vi "TCP - Client.vi"() -> ()   [LabVIEW 2023]
doc: "Demonstrates how to open a connection to an TCP server, read the data being sent, and display the data on a chart. This VI is designed to stop if the TCP connection is terminated."
panel:
  out "X4":bool
  out "X2":bool
  out "X3":bool
  out "X1":bool
  out "Switch 1":bool
  out "Switch 2":bool
  out "data out":string
  in  "Stop":bool
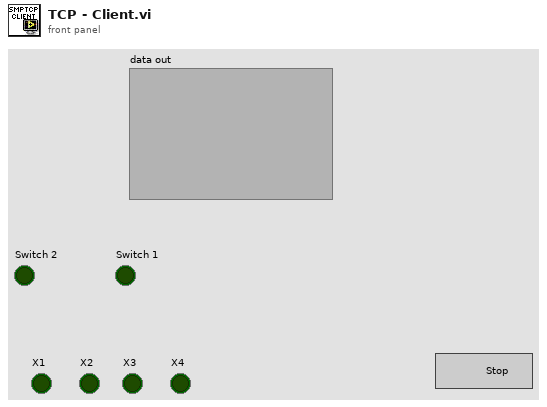
[diagram p1: front panel]
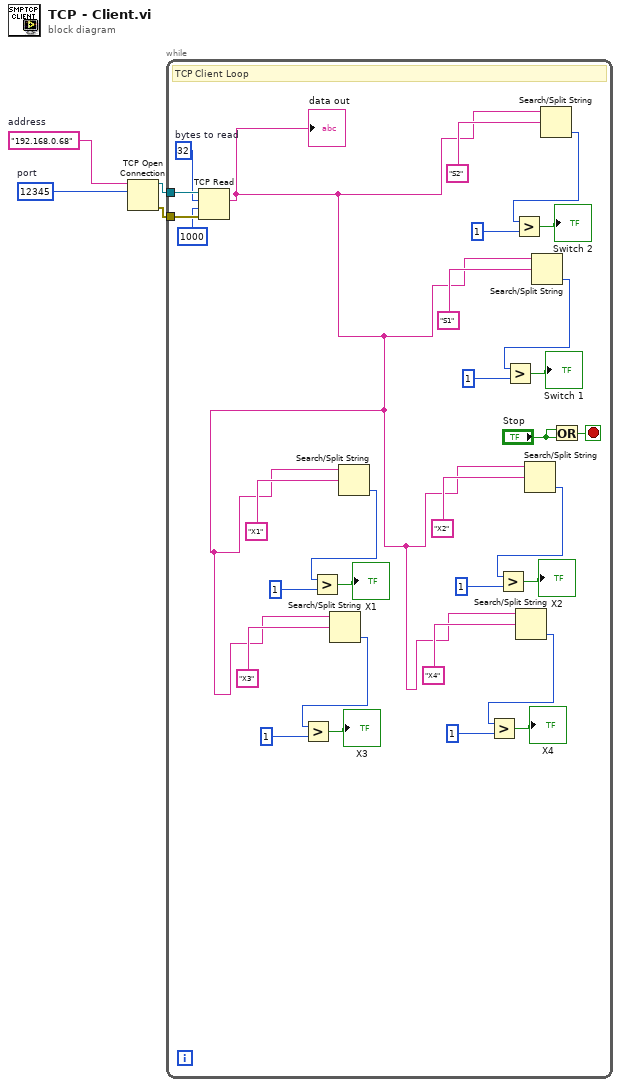
[diagram p0: block diagram]
diagram:
  w1 = u16 12345  # port
  w2 = "192.168.0.68"  # address
  n1 = TCP Open Connection(address=w2, remote port or service name=w1) -> (connection ID=w4:refnum<k5>, error out=w3:errorcluster)  [unwired: 3 in]
  n2 = while {
    tunnel: w3 -> [w34]
    tunnel: w4 -> [w35]
    stop <- w32 stop-if-true
    w33 = 32  # bytes to read
    # "TCP Client Loop"
    n3 = TCP Read(connection ID=w35, bytes to read=w33, error in (no error)=w34, 9:1000 ("timeout ms (25000)")) -> (data out=w5:string)  [unwired: 1 in, 2 out]
    "data out" <- w5
    n4 = Search/Split String(string=w5, search string/char (-)="X3" ("y")) -> (offset of match=w15:i32)  [unwired: 1 in, 2 out]
    n5 = Greater?(x=w15, y=1) -> (0:→"X3":bool)
    n6 = Search/Split String(string=w5, search string/char (-)="X1" ("y")) -> (offset of match=w19:i32)  [unwired: 1 in, 2 out]
    n7 = Greater?(x=w19, y=1) -> (0:→"X1":bool)
    n8 = Search/Split String(string=w5, search string/char (-)="X4" ("y")) -> (offset of match=w7:i32)  [unwired: 1 in, 2 out]
    n9 = Greater?(x=w7, y=1) -> (0:→"X4":bool)
    n10 = Search/Split String(string=w5, search string/char (-)="X2" ("y")) -> (offset of match=w11:i32)  [unwired: 1 in, 2 out]
    n11 = Greater?(x=w11, y=1) -> (0:→"X2":bool)
    n12 = Search/Split String(string=w5, search string/char (-)="S1" ("y")) -> (offset of match=w23:i32)  [unwired: 1 in, 2 out]
    n13 = Greater?(x=w23, y=1) -> (0:→"Switch 1":bool)
    n14 = Search/Split String(string=w5, search string/char (-)="S2" ("y")) -> (offset of match=w27:i32)  [unwired: 1 in, 2 out]
    n15 = Greater?(x=w27, y=1) -> (0:→"Switch 2":bool)
    n16 = Or(x="Stop", y="Stop") -> (x .or. y?=w32:bool)
  }
